vi "Controller Prepare Bumpless Transition Filter.vi"(10 "den in":dbl[](array[numeric]), 11 "num in":dbl[](array[numeric])) -> (1 "gain correction":dbl, 2 "den out":dbl[](array[numeric]), 3 "num out":dbl[](array[numeric]))   [LabVIEW 2011, in "Controller VIs.lvlib"]
uses:
  Controller VIs.lvlib
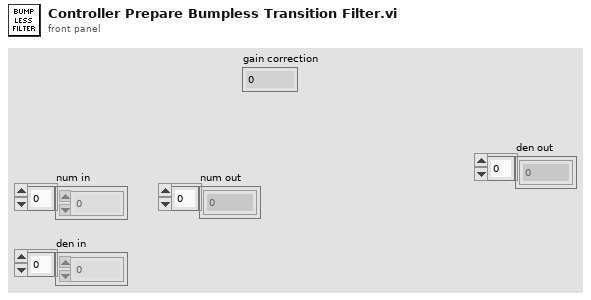
[diagram p1: front panel]
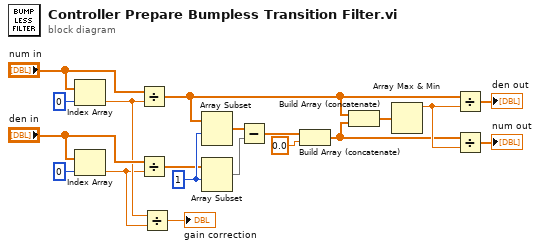
[diagram p0: block diagram]
diagram:
  w19 = 1 ("index")
  n1 = Index Array(array="num in", index=0) -> (element=w2:dbl)
  n2 = Index Array(array="den in", index=0) -> (element=w1:dbl)
  n3 = Divide(x="num in", y=w2) -> (x/y=w8:dbl[])
  n4 = Divide(x="den in", y=w1) -> (x/y=w10:dbl[])
  n5 = Divide(x=w2, y=w1) -> (x/y=→"gain correction":dbl)
  n6 = Array Subset(array=w8, index=w19) -> (w17:dbl[])  [unwired: 1 in]
  n7 = Array Subset(array=w10, index=w19) -> (w18:dbl[])  [unwired: 1 in]
  n8 = Subtract(x=w17, y=w18) -> (x-y=w15:dbl[])
  n9 = Build Array (concatenate)(w15, 0.0 ("Numeric")) -> (w6:dbl[])
  n10 = Build Array (concatenate)(w8, w6) -> (w9:dbl[])
  n11 = Array Max & Min(array=w9) -> (max value=w7:dbl)  [unwired: 3 out]
  n12 = Divide(x=w8, y=w7) -> (x/y=→"den out":dbl[])
  n13 = Divide(x=w6, y=w7) -> (x/y=→"num out":dbl[])
